vi "GetJointPosition.vi"(0 "error in (no error)":errorcluster, 9 "HighSpeedEServer":refnum<k24>) -> (4 "error out":errorcluster, 6 "Axes":i32[](array[numeric]), 8 "RCONF":i32, 10 "ToolNumber":i32, 15 "UserCoordinateNumber":i32)   [LabVIEW 2024, in "UnderAutomation.Yaskawa.lvlib"]
uses:
  UnderAutomation.Yaskawa.lvlib
  C:/Users/fg/Documents/Yaskawa.vi/LabVIEW_2024/UnderAutomation.Yaskawa/lib/UnderAutomation.Yaskawa.dll
  lib/UnderAutomation.Yaskawa.dll
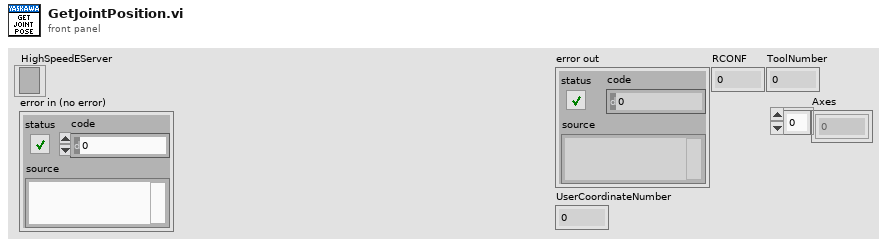
[diagram p1: front panel]
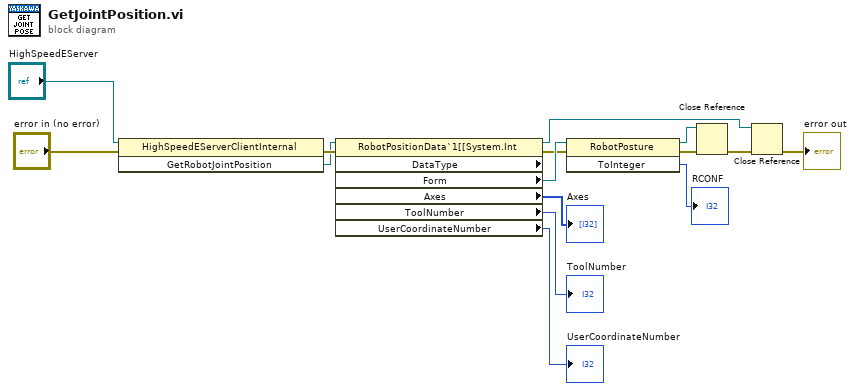
[diagram p0: block diagram]
diagram:
  n1 = invoke class="HighSpeedEServerClientInternal" method="GetRobotJointPosition"(reference="HighSpeedEServer", error in="error in (no error)") -> (error out=w13:errorcluster, "GetRobotJointPosition"=w12:refnum<k24>)  [unwired: 1 in, 1 out]
  n2 = property class="RobotPositionData`1[[System.Int" props=["DataType", "Form", "Axes", "ToolNumber", "UserCoordinateNumber"](reference=w12, error in=w13) -> (reference out=w1:refnum<k24>, error out=w10:errorcluster, "Form"=w11:refnum<k24>, "Axes"=→"Axes":i32[], "ToolNumber"=→"ToolNumber":i32, "UserCoordinateNumber"=→"UserCoordinateNumber":i32)  [unwired: 1 out]
  n3 = invoke class="RobotPosture" method="ToInteger"(reference=w11, error in=w10) -> (reference out=w2:refnum<k24>, error out=w3:errorcluster, "ToInteger"=→"RCONF":i32)  [unwired: 1 in]
  n4 = Close Reference(reference=w2, error in (no error)=w3) -> (error out=w5:errorcluster)
  n5 = Close Reference(reference=w1, error in (no error)=w5) -> (error out=→"error out":errorcluster)
